vi "Add Database RTM.vi"(8 "error in":errorcluster, 11 "Node Ptr":T3 format="%.0x") -> (0 "error out":errorcluster)   [LabVIEW 2020, in "Ballard ARINC 429 System Explorer.lvlib" / "Implementation.lvlib"]
doc: "This VI runs when the Add Database run-time menu is chosen. It allows the user to choose a database file and rename the database if they want a name other than the file name."
uses:
  Implementation.lvlib
  <vilib>/NI VeriStand/Custom Device Tools/Custom Device Utility Library/Custom Device Utility Library.lvlib
  Scripting/Ballard ARINC 429 Scripting.lvlib
  Scripting/Constants.vi
  Types/Path Control.ctl
  <vilib>/NI VeriStand/Custom Device API/Custom Device Item Ref.ctl
  <vilib>/NI VeriStand/Custom Device API/Custom Device API.lvlib
  Types/Browse Button.ctl
panel:
  in  "Path":T1
  in  "Database Name":string
  in  "Help":bool
  in  "Cancel":bool
  in  "OK":bool
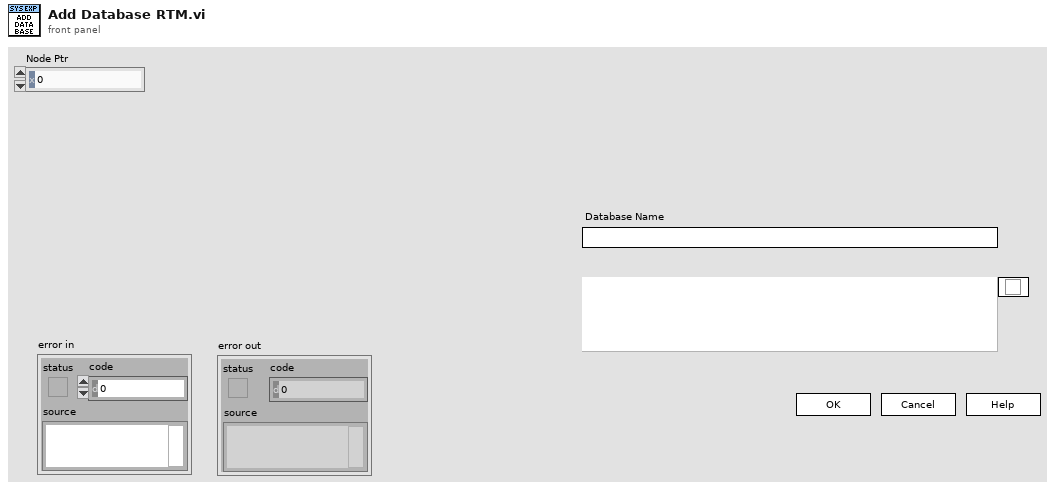
[diagram p1: front panel]
types:
  T1 = typedef "Ballard ARINC 429 System Explorer.lvlib/Implementation.lvlib/Path Control.ctl" = cluster{"file path":path, "Browse":T2}
  T2 = typedef "Ballard ARINC 429 System Explorer.lvlib/Implementation.lvlib/Browse Button.ctl" = bool
  T3 = typedef "Custom Device API.lvlib/Custom Device Item Ref.ctl" = u64
  T4 = cluster{"Database Name":string, "Database Path":path, "Node Ptr":T3}
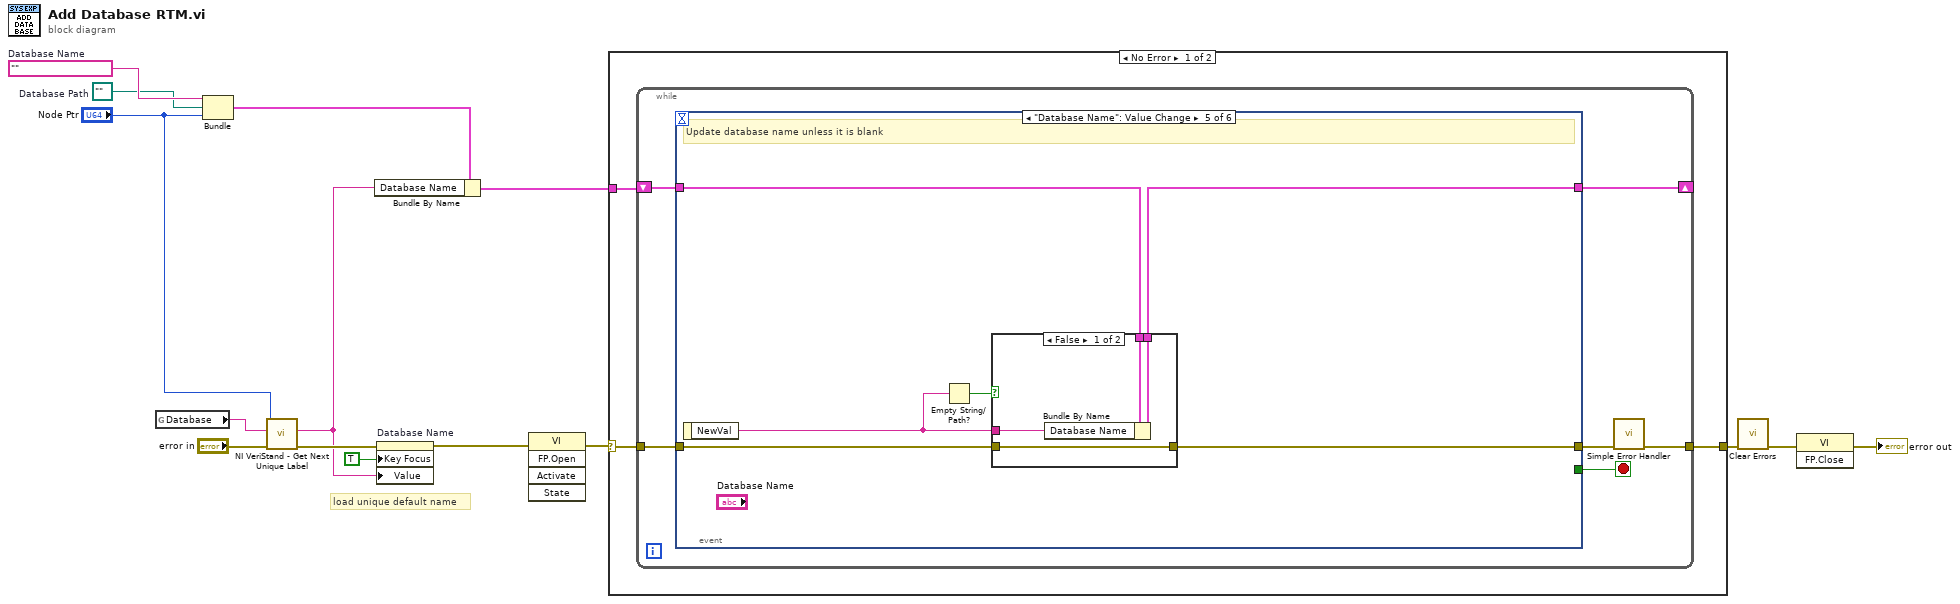
[diagram p0: block diagram]
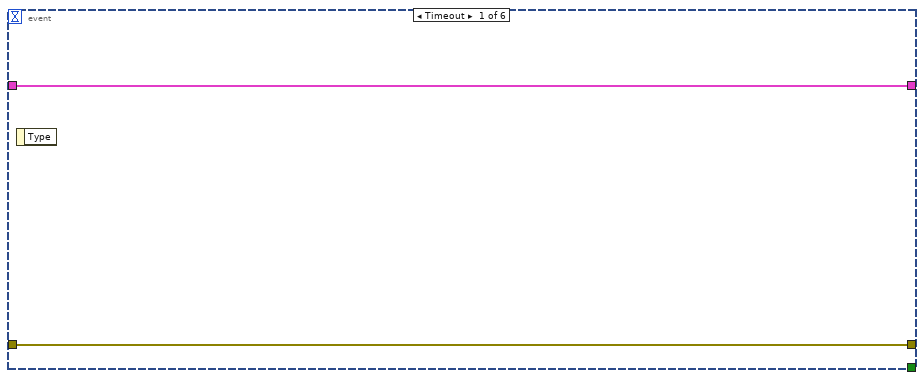
[diagram p2: hidden frame]
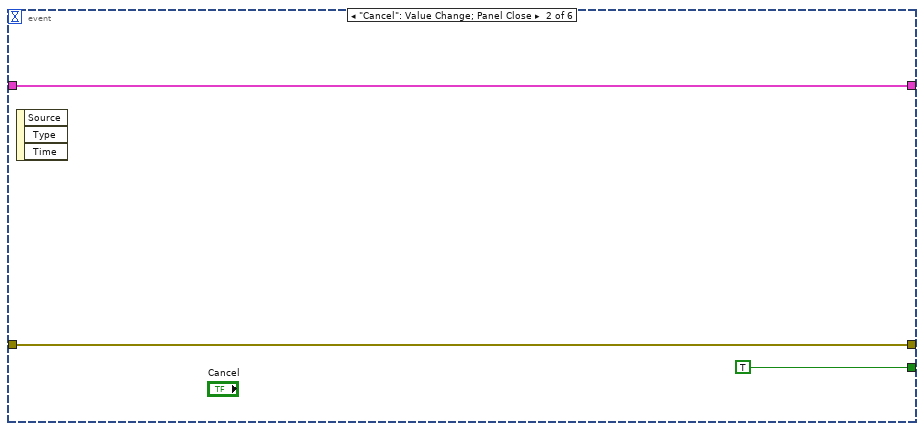
[diagram p3: hidden frame]
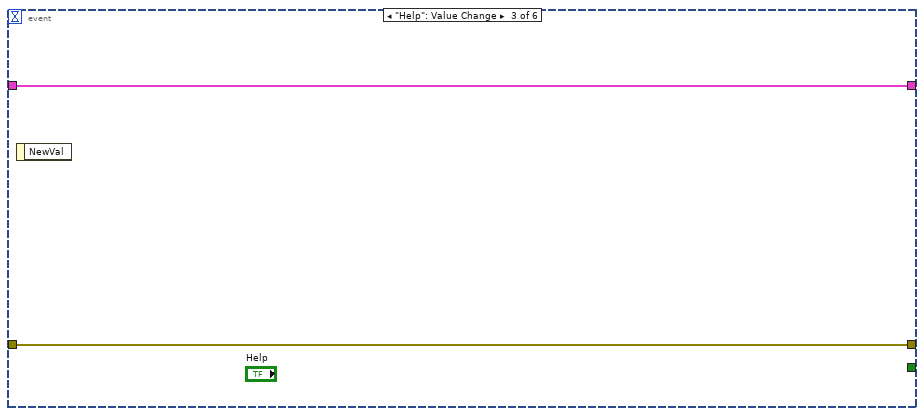
[diagram p4: hidden frame]
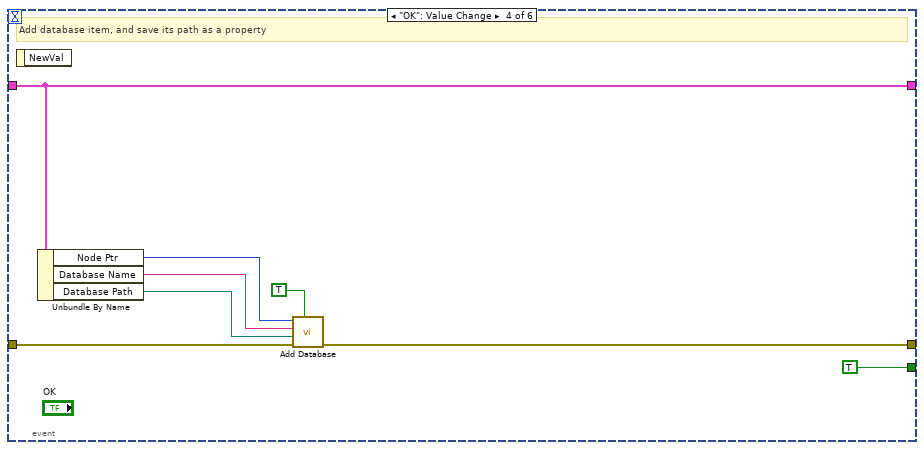
[diagram p5: hidden frame]
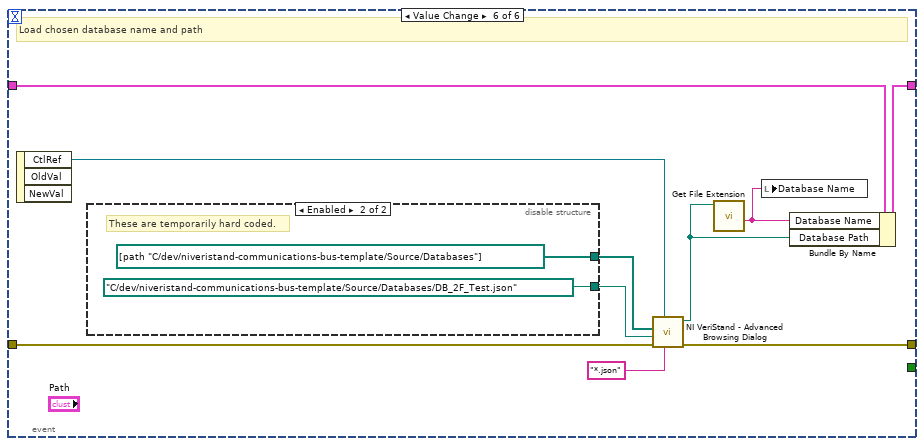
[diagram p7: hidden frame]
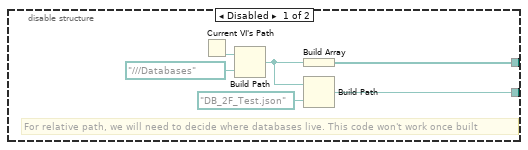
[diagram p8: hidden frame]
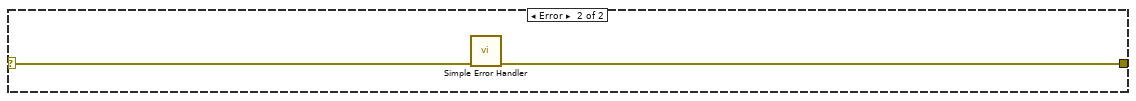
[diagram p9: hidden frame]
diagram:
  w1 = path ""  # Database Path
  w2 = ""  # Database Name
  # "load unique default name"
  n1 = global read "Constants.vi" "Database"() -> (w5:string)
  n2 = Bundle("Database Name"=w2, "Database Path"=w1, "Node Ptr"="Node Ptr") -> (w4:T4)  [unwired: 1 in]
  n3 = call <vilib>:"NI VeriStand - Get Next Unique Label.vi"("error in (no error)"="error in", "Label"=w5, "Parent Ref in"="Node Ptr") -> ("error out"=w7:errorcluster, "Label out"=w6:string)  [unwired: 5 in, 2 out]
  n4 = Bundle By Name(cluster=w4, "Database Name"=w6) -> (w13:T4)
  n5 = property on="Database Name" class="Str"(error in=w7, "Key Focus"=TRUE, "Value"=w6) -> (error out=w12:errorcluster)  [unwired: 1 in, 1 out]
  n6 = invoke class="VI" method="FP.Open"(error in=w12) -> (error out=w11:errorcluster)  [unwired: 4 in, 4 out]
  n7 = case shown="No Error" w11 {
    selector: w11 -> [w18 w71]
    tunnel: [w17 w70] -> w14
    tunnel: w13 -> [w16 _]
    frame No Error {
      n8 = while {
        tunnel: w18 -> [w24]
        tunnel: [w22] -> w17
        shift-right: [w19] -> _
        shift-left: w16 -> [w20]
        stop <- w21 stop-if-true
        n9 = event shown="[4] \"Database Name\": Value Change" {
          selector: _ -> [_ _ _ _ _ _]
          dyn-events: _ -> [_ _ _ _ _ _]
          timeout: _ -> [_ _ _ _ _ _]
          tunnel: [w26 w28 w31 w36 w44 w58] -> w23
          tunnel: w24 -> [w26 w28 w31 w38 w45 w60]
          tunnel: [_ TRUE ("Discard?") _ TRUE ("Discard?") _ _] -> w21
          tunnel: w20 -> [w25 w27 w30 w37 w41 w56]
          tunnel: [w25 w27 w30 w37 w40 w57] -> w19
          event Timeout {
            n10 = event-data() -> ()  [unwired: 1 in, 1 out]
          }
          event "Cancel": Value Change; Panel Close {
            n11 = event-data() -> ()  [unwired: 1 in, 3 out]
          }
          event "Help": Value Change {
            n12 = event-data() -> ()  [unwired: 1 in, 1 out]
          }
          event "OK": Value Change {
            # "Add database item, and save its path as a property"
            n13 = event-data() -> ()  [unwired: 1 in, 1 out]
            n14 = Unbundle By Name(w37) -> ("Node Ptr"=w35:T3, "Database Name"=w34:string, "Database Path"=w32:path)
            n15 = call "Add Database.vi"("Highlight? (F)"=TRUE, "error in"=w38, "Path"=w32, "Name"=w34, "Database section Ref"=w35) -> ("error out"=w36:errorcluster)  [unwired: 5 in, 1 out]
          }
          event "Database Name": Value Change {
            # "Update database name unless it is blank"
            n16 = event-data() -> ("NewVal"=w42:string)  [unwired: 1 in]
            n17 = Empty String/Path?(string/path=w42) -> (empty?=w43:bool)
            n18 = case shown="False" w43 {
              tunnel: w45 -> [w49 w51]
              tunnel: w42 -> [w47 _]
              tunnel: [w49 w51] -> w44
              tunnel: w41 -> [w48 w50]
              tunnel: [w46 w50] -> w40
              frame False {
                n19 = Bundle By Name(cluster=w48, "Database Name"=w47) -> (w46:T4)
              }
              frame True {
              }
            }
          }
          event Value Change {
            # "Load chosen database name and path"
            n20 = event-data() -> ("CtlRef"=w61:refnum<vi>)  [unwired: 1 in, 2 out]
            n21 = disable-structure shown="Enabled" {
              disable-tunnel: [w65 path[] [path "C:/dev/niveristand-communications-bus-template/Source/Databases"]] -> w53
              disable-tunnel: [w63 path "C:/dev/niveristand-communications-bus-template/Source/Databases/DB_2F_Test.json" ("Most recent path")] -> w52
              frame Disabled {
                # "For relative path, we will need to decide where databases live. This code won't work once built"
                n22 = Current VI's Path() -> (path=w67:path)
                n23 = Build Path(base path=w67, name or relative path=path "../../../Databases") -> (appended path=w64:path)
                n24 = Build Array(w64) -> (w65:path[])
                n25 = Build Path(base path=w64, name or relative path=path "DB_2F_Test.json") -> (appended path=w63:path)
              }
              frame Enabled {
                # "These are temporarily hard coded."
              }
            }
            n26 = call <vilib>:"NI VeriStand - Advanced Browsing Dialog.vi"("File Pattern"="*.json", "CtlRef"=w61, "error in (no error)"=w60, "Most recent path"=w52, "Paths"=w53) -> ("error out"=w58:errorcluster, "Selected file"=w54:path)  [unwired: 3 in, 2 out]
            n27 = call <vilib>:"Get File Extension.vi"("file"=w54) -> ("filename without extension"=w55:string)  [unwired: 6 in, 4 out]
            n28 = local write "Database Name"(w55) -> ()
            n29 = Bundle By Name(cluster=w56, "Database Name"=w55, "Database Path"=w54) -> (w57:T4)
          }
        }
        n30 = call <vilib>:"Simple Error Handler.vi"("error in (no error)"=w23) -> ("error out"=w22:errorcluster)  [unwired: 4 in, 4 out]
      }
    }
    frame Error {
      n31 = call <vilib>:"Simple Error Handler.vi"("error in (no error)"=w71) -> ("error out"=w70:errorcluster)  [unwired: 4 in, 4 out]
    }
  }
  n32 = call <vilib>:"Clear Errors.vi"("error in (no error)"=w14) -> ("error out"=w10:errorcluster)  [unwired: 5 in, 1 out]
  n33 = invoke class="VI" method="FP.Close"(error in=w10) -> (error out=→"error out":errorcluster)  [unwired: 2 in, 2 out]
